vi "son-FPGA_of Tank 1.vi"(3 "Port9/DIO8":bool, 4 "error out":errorcluster) -> ()   [LabVIEW 2012]
uses:
  <vilib>/rvi/interface/nirviReadWriteControl/nirviReadWriteControl.xnode
  <vilib>/rvi/interface/Simulation/niFpgaSimulationCallBeginRW.vi
  <vilib>/rvi/errors/niLvFpgaAdjustHostInterfaceError.vi
  NiFpgaLv.dll
  <vilib>/Utility/error.llb/Error Cluster From Error Code.vi
  <vilib>/rvi/interface/nirviCloseFPGA/nirviCloseFPGA.xnode
  <vilib>/FPGAPlugInAG/Dynamic/niLvFpga_Close_Dynamic.vi
  <vilib>/rvi/interface/nirviOpenFPGA/nirviOpenFPGA.xnode
  FPGA Bitfiles/mainframe_FPGATarget_FPGA-conrolofTan_KuVWLCbSiUA.lvbitx
  FPGA-conrol_of Tank1.vi
  <vilib>/FPGAPlugInAG/sbRIO-9632/niLvFpga_Open_sbRIO-9632.vi
  <vilib>/rvi/interface/common/dynamic/niFpgaDynamicAddResources.vi
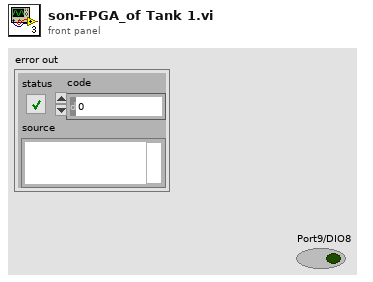
[diagram p1: front panel]
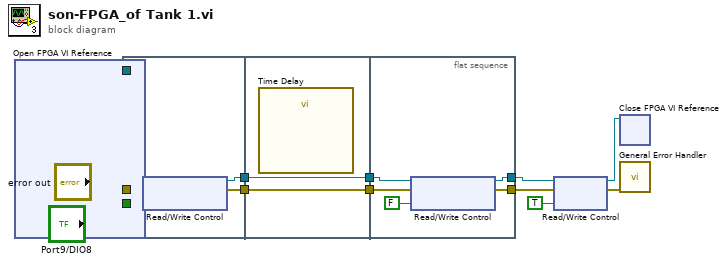
[diagram p0: block diagram]
diagram:
  n1 = xnode "Open FPGA VI Reference"() -> ("FPGA VI Reference Out"=w1:refnum<k20>)  [unwired: 2 in, 1 out]
  n2 = flat-sequence {
    tunnel: w1 -> [w17]
    tunnel: "error out" -> [w15]
    tunnel: "Port9/DIO8" -> [w13]
    tunnel: [w16] -> w11
    tunnel: [w14] -> w10
    tunnel: w11 -> [w19]
    tunnel: w10 -> [w18]
    tunnel: [w19] -> w9
    tunnel: [w18] -> w8
    tunnel: w9 -> [w24]
    tunnel: w8 -> [w22]
    tunnel: [w23] -> w6
    tunnel: [w21] -> w5
    frame #0 {
      n3 = xnode "Read/Write Control"("FPGA VI Reference In"=w17, "error in"=w15, "Port9/DIO8"=w13) -> ("FPGA VI Reference Out"=w16:refnum<k20>, "error out"=w14:errorcluster)
    }
    frame #1 {
      n4 = call "Time Delay"() -> ()  [unwired: 11 in, 1 out]
    }
    frame #2 {
      n5 = xnode "Read/Write Control"("FPGA VI Reference In"=w24, "error in"=w22, "Port9/DIO8"=FALSE) -> ("FPGA VI Reference Out"=w23:refnum<k20>, "error out"=w21:errorcluster)
    }
  }
  n6 = xnode "Read/Write Control"("FPGA VI Reference In"=w6, "error in"=w5, "stop"=TRUE) -> ("FPGA VI Reference Out"=w3:refnum<k20>, "error out"=w2:errorcluster)
  n7 = xnode "Close FPGA VI Reference"("FPGA VI Reference In"=w3) -> ()  [unwired: 1 in, 1 out]
  n8 = call <vilib>:"General Error Handler.vi"("error in (no error)"=w2) -> ()  [unwired: 10 in, 5 out]
